vi "Send_outlook_mail_activex.vi"(5 "Attachments":path[](array[path]), 6 "CC":string, 7 "Importance":i32(ring)=1 items=["Low", "Normal", "High"], 8 "error in":errorcluster, 9 "Message":string, 10 "Subject":string, 11 "To":string) -> (0 "error out":errorcluster)   [LabVIEW 2018]
doc: "This example uses Microsoft Outlook activeX objects to create a new message and then send that message using the Microsoft Outlook engine. The VI was developed and testing using Microsoft Outlook 2002, but most version of Microsoft Outlook should be compatible with the program.\n\nEnter data into the To, Subject, and message controls on the front panel. The other controls, CC and BCC, are optional. When using multiple email addresses separate addresses with a semicolon. \n\nRun the VI to send an email to the specified email address. If you have the E-mail security update installed with Microsoft Outlook 2002, you will be prompted to authorize the automated email and override the security warning. Click OK in the message box to send the email.\n\nNote: \nFor truly automated messaging, you can override this warning message programmatically using third party software."
panel:
  in  "BCC":string
  in  "Outlook._MailItem":refnum<k7>
  in  "Outlook._Application":refnum<k7>
  # "Select Help»Show Context Help and move the cursor over the VI icon to display help for this VI."
  # "Sending E-Mail with MS Outlook Using ActiveX"
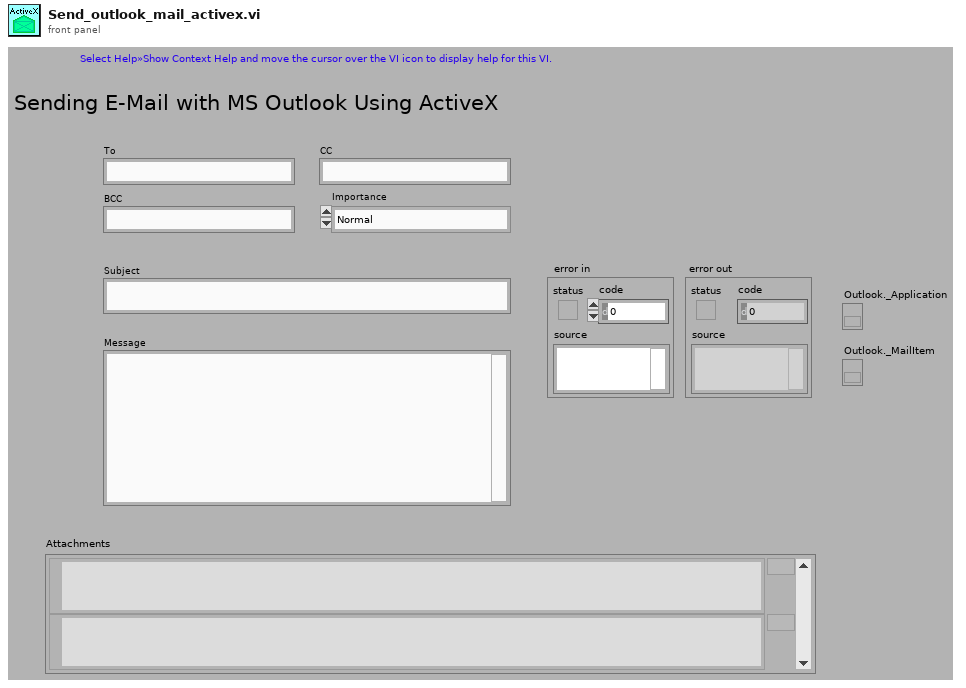
[diagram p1: front panel]
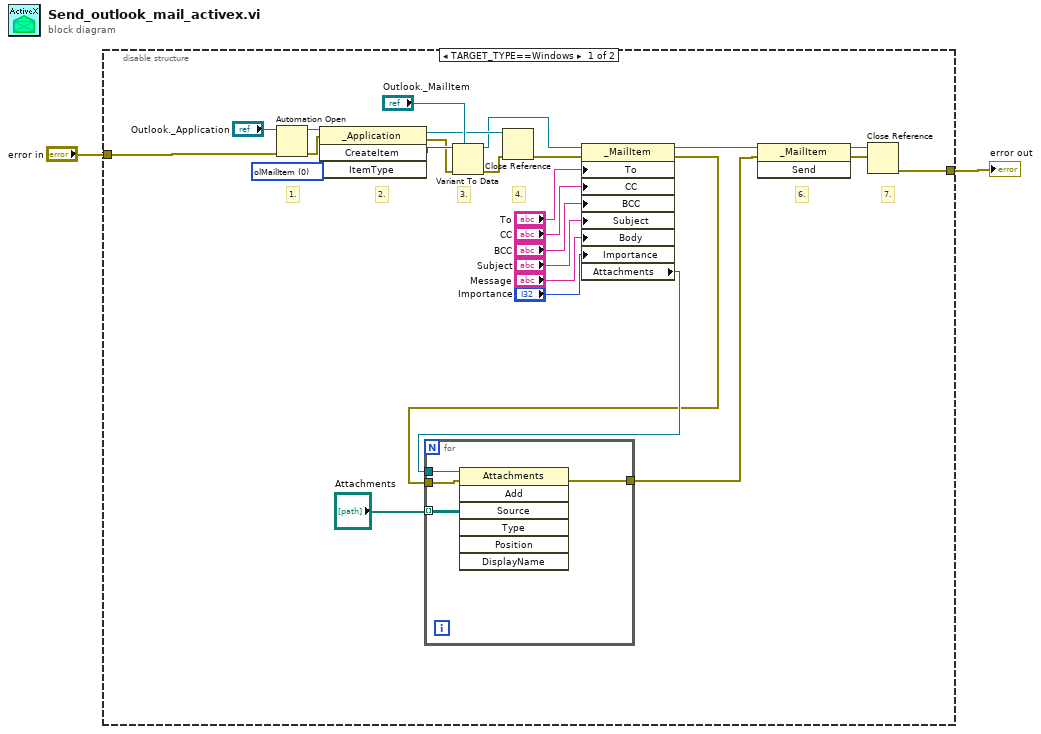
[diagram p0: block diagram]
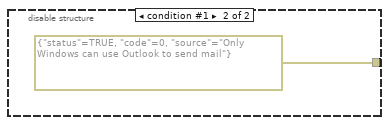
[diagram p2: hidden frame]
diagram:
  n1 = disable-structure shown="TARGET_TYPE==Windows" {
    disable-tunnel: "error in" -> [w17 _]
    disable-tunnel: [w13 errorcluster {"status"=TRUE, "code"=0, "source"="Only Windows can use Outlook to send mail"} ("error out")] -> w1
    frame condition #0 (active) {
      w26 = 0 items=["olMailItem", "olAppointmentItem", "olContactItem", "olTaskItem", "olJournalItem", "olNoteItem", "olPostItem"] ("ItemType")
      # "7."
      # "6."
      # "4."
      # "3."
      # "2."
      # "1."
      n2 = Automation Open(error in (no error)=w17, Automation Refnum="Outlook._Application") -> (Automation Refnum=w27:refnum<k7>, error out=w18:errorcluster)  [unwired: 2 in]
      n3 = invoke class="_Application" method="CreateItem"(reference=w27, error in=w18, "ItemType"=w26) -> (reference out=w22:refnum<k7>, error out=w16:errorcluster, "CreateItem"=w25:variant)  [unwired: 1 in, 1 out]
      n4 = Variant To Data(error in=w16, type="Outlook._MailItem", Variant=w25) -> (data=w21:refnum<k7>, error out=w15:errorcluster)
      n5 = Close Reference(reference=w22, error in (no error)=w15) -> (error out=w14:errorcluster)
      n6 = property class="_MailItem"(reference=w21, error in=w14, "To"="To", "CC"="CC", "BCC"="BCC", "Subject"="Subject", "Body"="Message", "Importance"="Importance") -> (reference out=w3:refnum<k7>, error out=w5:errorcluster, "Attachments"=w7:refnum<k7>)
      n7 = for {
        tunnel: w7 -> [w32]
        tunnel: "Attachments" -> [w31] mode=indexing
        tunnel: w5 -> [w30]
        tunnel: [w29] -> w4
        n8 = invoke class="Attachments" method="Add"(reference=w32, error in=w30, "Source"=w31) -> (error out=w29:errorcluster)  [unwired: 4 in, 6 out]
      }
      n9 = invoke class="_MailItem" method="Send"(reference=w3, error in=w4) -> (reference out=w20:refnum<k7>, error out=w19:errorcluster)  [unwired: 1 in, 1 out]
      n10 = Close Reference(reference=w20, error in (no error)=w19) -> (error out=w13:errorcluster)
    }
    frame condition #1 {
    }
  }
  "error out" <- w1
